vi "RRTPlan.vi"(8 "Initial Pos x,y":dbl[](array[numeric]), 9 "Dest x,y":dbl[](array[numeric]), 10 "IA State":T3={"our_robots"=[], "enemy_robots"=[], "balls"=[], "geometry"={"field_length"=0, "field_width"=0, "goal_width"=0, "goal_depth"=0, "center_circle_radius"=0, "defense_width"=0, "defense_depth"=0, "free_kick_from_defense_dist"=0, "penalty_spot_from_field_line_dist"=0, "penalty_line_from_spot_dist"=0, "half_moon_depth"=0, "half_moon_width"=0}, "IA Judge"={"stage"="", "command"="", "our_goalie_id"=0.0, "enemy_goalie_id"=0.0, "command enum"=enum."Halt", "Time"=enum."Azul"}, "Received Timestamp"=timestamp(0 s since 1904-01-01), "Events"={"Touch"=FALSE, "id touch"=0.0, "Ball out of \nVision"=FALSE, "Ball inside \nGoalie area"=FALSE, "Robot not responding"=FALSE, "Robots responding status"=[1.0, 1.0, 1.0, 1.0, 1.0, 1.0], "Enemy Ball \nPossession"=FALSE, "Id ini Possession"=0.0, "Ball Possesion"=FALSE, "Id Possesion"=0.0, "Ball at\nour goal side"=FALSE, "Ball at\ntouchline"=FALSE, "Ball at\nenemy goal side"=FALSE}}, 11 "Robot":T4={"id"=0, "function"=enum."Attacker", "x"=0.0, "y"=0.0, "orientation"=0.0, "v_tangent"=0.0, "v_normal"=0.0, "v_ang"=0.0, "kick_x"=0.0, "kick_z"=0.0, "dribble"=FALSE, "Timestamp"=timestamp(0 s since 1904-01-01), "estimatives"={"est_v_tangent"=0.0, "est_v_normal"=0.0, "est_vx"=0.0, "est_vy"=0.0, "Pos Robot Est"=[]}, "dest_x_kick"=0.0, "dest_y_kick"=0.0, "Gap Coord"=[], "States"=enum."GoToTangent", "Path "=[], "Path  Smooth"=[], "Dest"=[]}) -> (0 "Path":dbl[][](array[numeric]), 1 "Smooth Path":dbl[][](array[numeric]))   [LabVIEW 2018]
uses:
  Core/AI Robot.ctl
  Intel/Functions Enum.ctl
  Intel/AttackerStates.ctl
  PathDests.ctl
  PathDest.ctl
  Core/AI Input.ctl
  Core/AI Ball.ctl
  Core/Field Size.ctl
  Core/AI Judge.ctl
  Intel/Command Enum.ctl
  Util/Events/Events.ctl
  kD-tree/KD-Tree.ctl
  kD-tree/Node.ctl
  <vilib>/Analysis/_algsub.llb/Real Vector Norm.vi
  <vilib>/Analysis/NI_AALPro.lvlib
panel:
  out "New KD-Tree":T1
  out "x > y? 2":bool
  out "Modulo":dbl
  in  "WayPointProb":dbl=0.6 format="%#_13g"
  in  "GoalProb":dbl=0.1 format="%#_13g"
  in  "Step":dbl=80.0
  out "Elapsed Time (s)":dbl
  out "Time has Elapsed":bool
  in  "threshold":dbl=80.0
  out "Goal":dbl[](array[numeric])
  out "Initial State":dbl[](array[numeric])
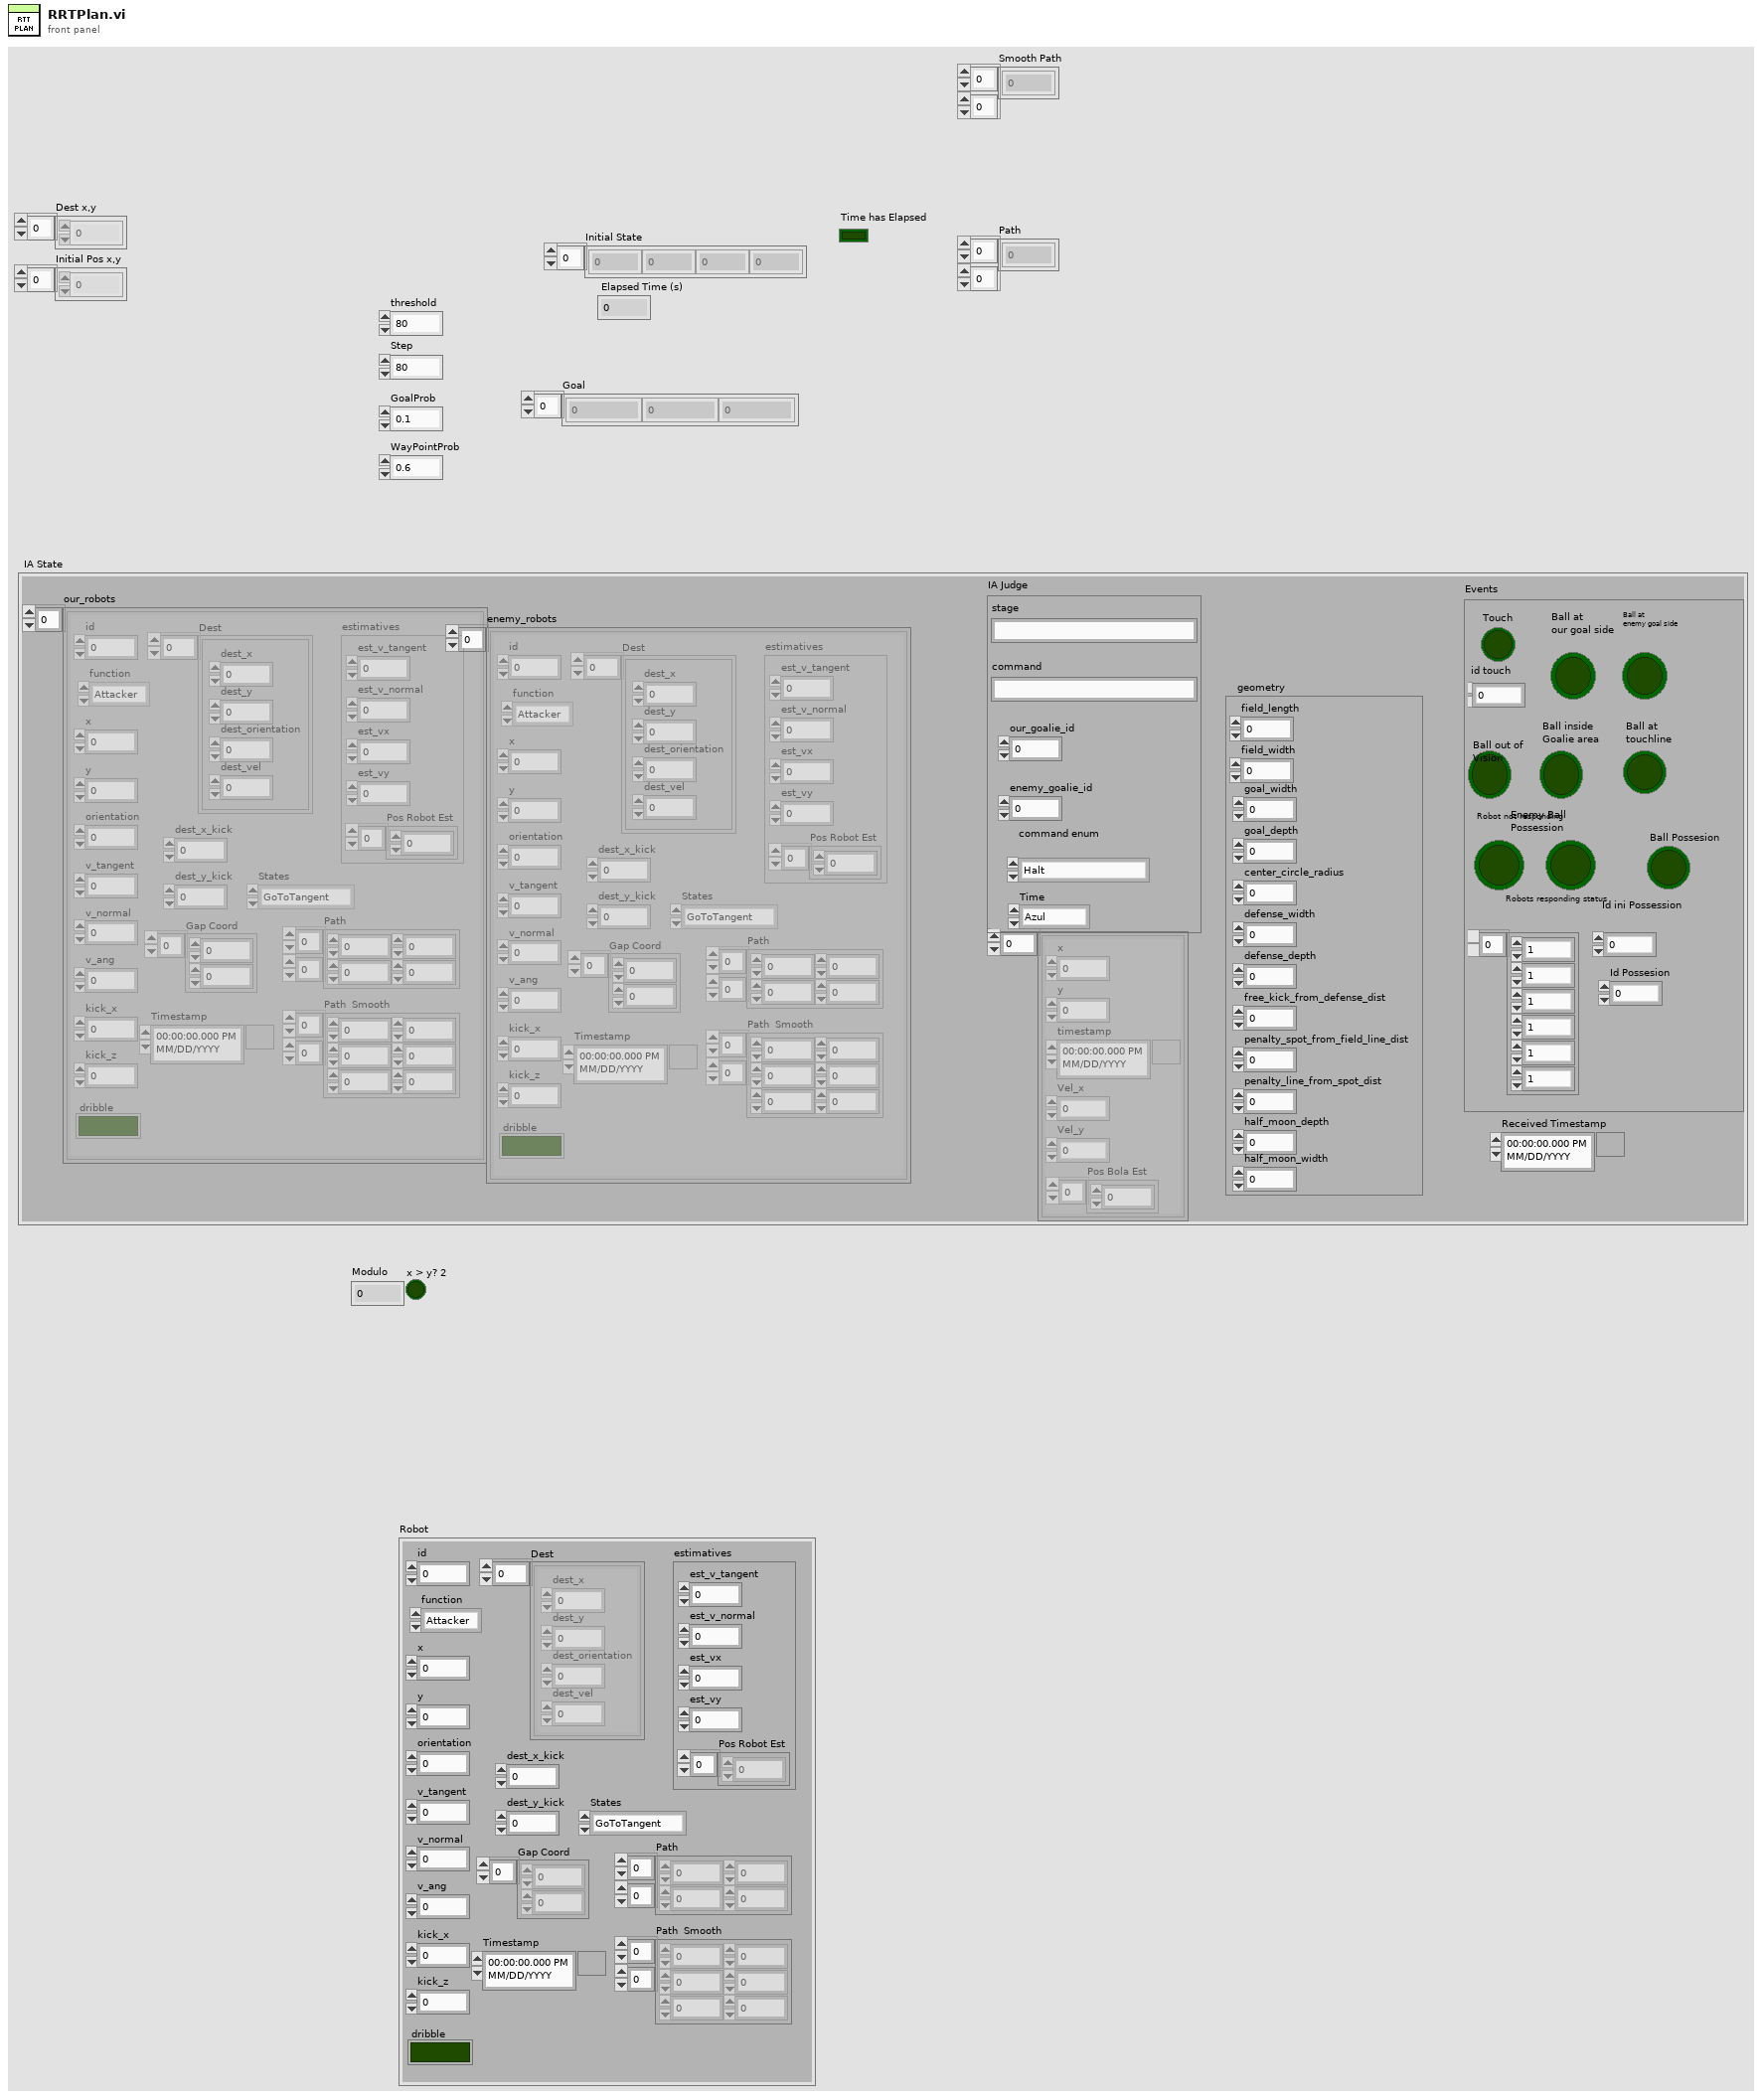
[diagram p1: front panel]
types:
  T1 = typedef "KD-Tree.ctl" = T2[]
  T2 = typedef "Node.ctl" = cluster{"axis":enum16{"null", "x", "y"}, "value":dbl, "left":dbl, "right":dbl, "Point":dbl[]}
  T3 = typedef "AI Input.ctl" = cluster{"our_robots":T4[], "enemy_robots":T4[], "balls":T9[], "geometry":T10, "IA Judge":T11, "Received Timestamp":timestamp, "Events":T13}
  T4 = typedef "AI Robot.ctl" = cluster{"id":u32, "function":T5, "x":dbl, "y":dbl, "orientation":dbl, "v_tangent":dbl, "v_normal":dbl, "v_ang":dbl, "kick_x":dbl, "kick_z":dbl, "dribble":bool, "Timestamp":timestamp, "estimatives":cluster{"est_v_tangent":dbl, "est_v_normal":dbl, "est_vx":dbl, "est_vy":dbl, "Pos Robot Est":dbl[]}, "dest_x_kick":dbl, "dest_y_kick":dbl, "Gap Coord":dbl[], "States":T6, "Path ":dbl[][], "Path  Smooth":dbl[][], "Dest":T7}
  T5 = typedef "Functions Enum.ctl" = enum16{"Attacker", "Goalie", "Defender", "Striker", "Goto 0", "Dummy", "Kicker", "ZigZag"}
  T6 = typedef "AttackerStates.ctl" = enum16{"Pass", "GoToTangent", "BallGetting", "GoToKick", "Rotate anti-clockwise", "Rotate Clockwise", ""}
  T7 = typedef "PathDests.ctl" = T8[]
  T8 = typedef "PathDest.ctl" = cluster{"dest_x":dbl, "dest_y":dbl, "dest_orientation":dbl, "dest_vel":dbl}
  T9 = typedef "AI Ball.ctl" = cluster{"x":dbl, "y":dbl, "timestamp":timestamp, "Vel_x":dbl, "Vel_y":dbl, "Pos Bola Est":dbl[]}
  T10 = typedef "Field Size.ctl" = cluster{"field_length":u32, "field_width":u32, "goal_width":u32, "goal_depth":u32, "center_circle_radius":u32, "defense_width":u32, "defense_depth":u32, "free_kick_from_defense_dist":u32, "penalty_spot_from_field_line_dist":u32, "penalty_line_from_spot_dist":u32, "half_moon_depth":u32, "half_moon_width":u32}
  T11 = typedef "AI Judge.ctl" = cluster{"stage":string, "command":string, "our_goalie_id":dbl, "enemy_goalie_id":dbl, "command enum":T12, "Time":enum16{"Azul", "Amarelo"}}
  T12 = typedef "Command Enum.ctl" = enum16{"Halt", "Stop", "Force Start", "PKA Normal Start", "Prepare Kickoff Ally", "PKE Normal Start", "Prepare Kickoff Enemy", "Prepare Penalty Ally", "PPA Normal Start", "Prepare Penalty Enemy", "PPE Normal Start", "Ball Placement Enemy Up", "Ball Placement Enemy Down", "Ball Placement Ally Up", "Ball Placement Ally Mid", "Ball Placement Ally Down", "Indirect Free Enemy", "Indirect Free Ally", "Timeout Enemy", "Timeout Ally", "Goal Enemy", "Goal Ally", "Normal Half Time", "Extra Time Break", "Extra Half Time", "None", "Post Game"}
  T13 = typedef "Events.ctl" = cluster{"Touch":bool, "id touch":dbl, "Ball out of \nVision":bool, "Ball inside \nGoalie area":bool, "Robot not responding":bool, "Robots responding status":dbl[], "Enemy Ball \nPossession":bool, "Id ini Possession":dbl, "Ball Possesion":bool, "Id Possesion":dbl, "Ball at\nour goal side":bool, "Ball at\ntouchline":bool, "Ball at\nenemy goal side":bool}
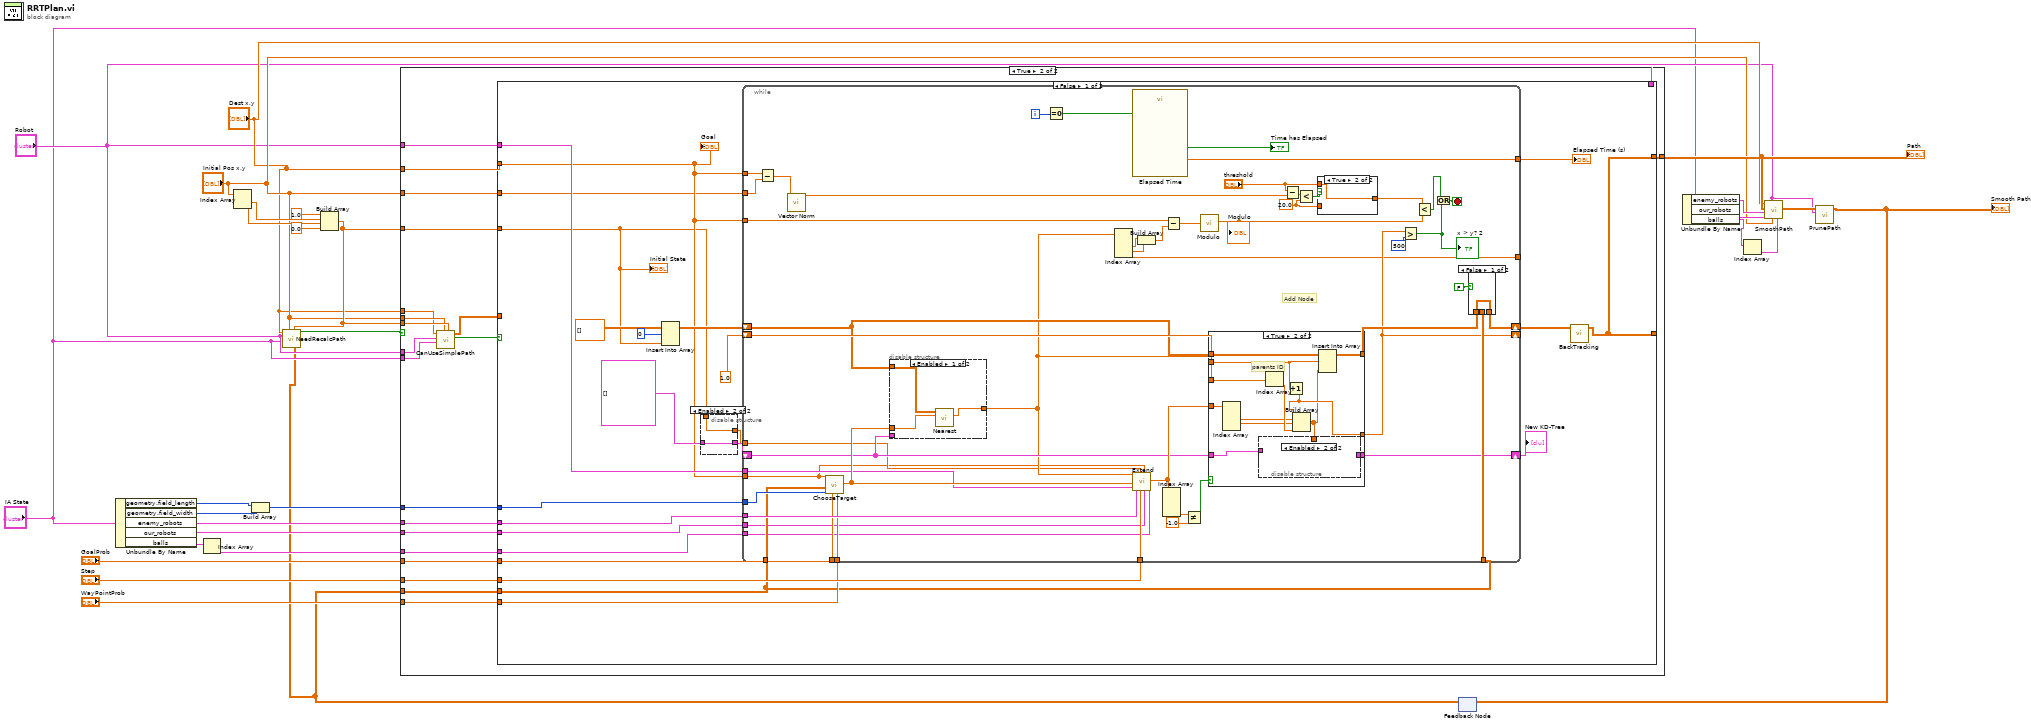
[diagram p0: block diagram]
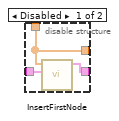
[diagram p3: hidden frame]
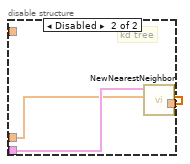
[diagram p4: hidden frame]
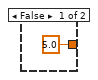
[diagram p5: hidden frame]
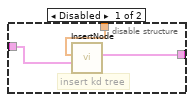
[diagram p8: hidden frame]
diagram:
  n1 = Unbundle By Name("IA State") -> ("geometry.field_length"=w28:u32, "geometry.field_width"=w27:u32, "enemy_robots"=w22:T4[], "our_robots"=w19:T4[], "balls"=w9:T9[])
  n2 = Index Array(array=w9) -> (element=w8:T9)  [unwired: 1 in]
  n3 = Index Array(array="Initial Pos x,y") -> (element #1=w18:dbl, element #2=w17:dbl)  [unwired: 2 in]
  n4 = Build Array(w28, w27) -> (w26:u32[])
  n5 = Build Array(1.0 ("element"), w18, w17, 0.0 ("element")) -> (w6:dbl[])
  n6 = feedback #1() -> (w1:dbl[][])  [unwired: 1 in]
  n7 = call "NeedRecalcPath.vi"("SmoothPath"=w1, "Initial State"=w6, "Pos x,y"="Initial Pos x,y", "IA State"="IA State", "Robot"="Robot", "Dest x,y"="Dest x,y") -> ("Boolean"=w7:bool)  [unwired: 5 in]
  n8 = case shown="True" w7 {
    tunnel: w26 -> [_ w49]
    tunnel: "Step" -> [_ w48]
    tunnel: "GoalProb" -> [_ w47]
    tunnel: "WayPointProb" -> [_ w46]
    tunnel: w22 -> [_ w45]
    tunnel: w6 -> [_ w44]
    tunnel: w1 -> [w29 w43]
    tunnel: w19 -> [_ w42]
    tunnel: [w29 w41] -> w14
    tunnel: "Dest x,y" -> [_ w40]
    tunnel: "Initial Pos x,y" -> [_ w39]
    tunnel: "Robot" -> [_ w38]
    tunnel: w8 -> [_ w37]
    tunnel: w6 -> [_ w36]
    tunnel: "Initial Pos x,y" -> [_ w35]
    tunnel: "Dest x,y" -> [_ w34]
    tunnel: "Robot" -> [_ w33]
    tunnel: "IA State" -> [_ w32]
    frame False {
    }
    frame True {
      n9 = call "CanUseSimplePath.vi"("Initial State"=w36, "Pos x,y"=w35, "IA State"=w32, "Robot"=w33, "Dest x,y"=w34) -> (2:"Simple Path"=w30:bool, 3:"Simple Path"=w31:dbl[][])  [unwired: 5 in]
      n10 = case shown="False" w30 {
        tunnel: w49 -> [w62 _]
        tunnel: w48 -> [w69 _]
        tunnel: w38 -> [w57 _]
        tunnel: w47 -> [w67 _]
        tunnel: w46 -> [w66 _]
        tunnel: w45 -> [w65 _]
        tunnel: w43 -> [w64 _]
        tunnel: [w55 w156] -> w41
        tunnel: w38 -> [_ _]
        tunnel: [w55 w156] -> _
        tunnel: w40 -> [w54 _]
        tunnel: w39 -> [w53 _]
        tunnel: w44 -> [w52 _]
        tunnel: w42 -> [w51 _]
        tunnel: w37 -> [w50 _]
        tunnel: w31 -> [_ w156]
        frame False {
          n11 = Insert Into Array(array=dbl[][] [] ("Pontos"), index (row)=0, new element=w52) -> (w70:dbl[][])  [unwired: 1 in]
          n12 = disable-structure shown="Enabled" {
            disable-tunnel: [w75 w77] -> w60
            disable-tunnel: T1 [] ("New KD-Tree") -> [w74 w77]
            disable-tunnel: w52 -> [w73 w76]
            disable-tunnel: [w73 w76] -> w56
            frame Disabled {
              n13 = call "InsertFirstNode.vi"("New KD-Tree in"=w74, "Tree"=w73) -> ("New KD-Tree out"=w75:T1)  [unwired: 9 in]
            }
            frame Enabled {
            }
          }
          n14 = while {
            tunnel: w54 -> [w126]
            tunnel: w54 -> [w81]
            tunnel: w62 -> [w123]
            shift-right: [w107] -> w63
            shift-left: w70 -> [w106]
            tunnel: w65 -> [w121]
            tunnel: w69 -> [w120]
            shift-right: [w103] -> _
            shift-left: 1.0 -> [w111]
            tunnel: w64 -> [w110]
            tunnel: w64 -> [w109]
            tunnel: w67 -> [w101]
            tunnel: w66 -> [w100]
            tunnel: [w97] -> _
            tunnel: w54 -> [w96]
            shift-right: [w89] -> w61
            shift-left: w60 -> [w88]
            tunnel: [w86] -> w58
            tunnel: w57 -> [w83]
            tunnel: w56 -> [w82]
            tunnel: w53 -> [w80]
            tunnel: w51 -> [w79]
            tunnel: w50 -> [w78]
            i -> [w85]
            stop <- w115 stop-if-true
            w90 = 20.0 ("y")
            # "Add Node"
            n15 = Subtract(x=w96, y=w80) -> (x-y=w95:dbl[])
            n16 = call-poly <vilib>:"Vector Norm.vi"("Input Vector"=w95) -> ("norm"=w93:dbl)  [unwired: 9 in, 1 out]
            n17 = call "ChooseTarget.vi"("WayPointProb"=w100, "GoalProb"=w101, "Field Geometry"=w123, "WayPointCache"=w110, "Goal"=w81) -> ("Target"=w122:dbl[])  [unwired: 6 in]
            n18 = disable-structure shown="Enabled" {
              disable-tunnel: w122 -> [w130 w132]
              disable-tunnel: w106 -> [w129 _]
              disable-tunnel: w88 -> [_ w133]
              disable-tunnel: [w128 w131] -> w87
              frame Enabled {
                n19 = call "Nearest.vi"("Target"=w130, "Pontos"=w129) -> ("Nearest"=w128:dbl[])  [unwired: 9 in]
              }
              frame Disabled {
                # "kd tree"
                n20 = call "NewNearestNeighbor.vi"("q"=w132, "KD-Tree"=w133) -> ("Nearest"=w131:dbl[])  [unwired: 9 in]
              }
            }
            n21 = Equal To 0?(x=w85) -> (x = 0?=w84:bool)
            n22 = Index Array(array=w87) -> (element #2=w114:dbl, element #3=w113:dbl, element #4=w97:dbl)  [unwired: 4 in, 1 out]
            n23 = call "Elapsed Time"("Auto Reset"=w84) -> ("Elapsed Time (s)"=w86:dbl, "Time has Elapsed"=→"Time has Elapsed":bool)  [unwired: 11 in, 6 out]
            n24 = call "Extend.vi"("Ball"=w78, "our_robots"=w79, "Goal"=w81, "Step"=w120, "Initial State"=w82, "enemy_robots"=w121, "Robot in"=w83, "Target"=w122, "Nearest"=w87) -> ("New State"=w116:dbl[])  [unwired: 2 in]
            n25 = Build Array(w114, w113) -> (w112:dbl[])
            n26 = Index Array(array=w116) -> (element #4=w119:dbl)  [unwired: 4 in, 3 out]
            n27 = Subtract(x=w126, y=w112) -> (x-y=w127:dbl[])
            n28 = Not Equal?(x=w119, y=-1.0) -> (x != y?=w117:bool)
            n29 = call "Modulo.vi"("2D vector"=w127) -> ("Modulo"=w125:dbl)  [unwired: 10 in]
            "Modulo" <- w125
            n30 = case shown="True" w117 {
              tunnel: w106 -> [w140 w152]
              tunnel: [w140 w148] -> w108
              tunnel: w116 -> [_ w151]
              tunnel: w111 -> [w139 w147]
              tunnel: w87 -> [_ w150]
              tunnel: [w139 w142] -> w103
              tunnel: [w138 w146] -> w89
              tunnel: w88 -> [w138 w145]
              frame False {
              }
              frame True {
                # "parents ID"
                n31 = Index Array(array=w151) -> (element #2=w144:dbl, element #3=w143:dbl)  [unwired: 4 in, 2 out]
                n32 = Index Array(array=w150) -> (element=w149:dbl)  [unwired: 1 in]
                n33 = Increment(x=w147) -> (x+1=w142:dbl)
                n34 = Build Array(w142, w144, w143, w149) -> (w141:dbl[])
                n35 = disable-structure shown="Enabled" {
                  disable-tunnel: [w155 _] -> w146
                  disable-tunnel: w145 -> [w154 _]
                  disable-tunnel: w141 -> [w153 _]
                  frame Disabled {
                    # "insert kd tree"
                    n36 = call "InsertNode.vi"("KD-Tree"=w154, "New Node"=w153) -> ("New KD-Tree"=w155:T1)  [unwired: 9 in]
                  }
                  frame Enabled {
                  }
                }
                n37 = Insert Into Array(array=w152, index (row)=w147, new element=w141) -> (w148:dbl[][])  [unwired: 1 in]
              }
            }
            n38 = Subtract(x="threshold", y=w93) -> (x-y=w91:dbl)
            n39 = Less?(x=w91, y=w90) -> (x < y?=w92:bool)
            n40 = case shown="True" w92 {
              tunnel: [5.0 ("threshold") w135] -> w124
              tunnel: "threshold" -> [_ w135]
              tunnel: w90 -> [_ _]
              frame False {
              }
              frame True {
              }
            }
            n41 = Greater?(x=w103, y=500) -> (0:w98:bool)
            "x > y? 2" <- w98
            n42 = Less?(x=w125, y=w124) -> (x < y?=w99:bool)
            n43 = Or(x=w99, y=w98) -> (x .or. y?=w115:bool)
            n44 = case shown="False" FALSE {
              tunnel: w109 -> [_ w137]
              tunnel: [w136 w137] -> w107
              tunnel: w108 -> [w136 _]
              frame False {
              }
              frame True {
              }
            }
          }
          "New KD-Tree" <- w61
          "Elapsed Time (s)" <- w58
          n45 = call "BackTracking.vi"("Pontos"=w63) -> ("Path"=w55:dbl[][])  [unwired: 9 in, 1 out]
          "Initial State" <- w52
          "Goal" <- w54
        }
        frame True {
        }
      }
    }
  }
  "Path" <- w14
  n46 = Unbundle By Name("IA State") -> ("enemy_robots"=w15:T4[], "our_robots"=w16:T4[], "balls"=w11:T9[])
  n47 = Index Array(array=w11) -> (element=w10:T9)  [unwired: 1 in]
  n48 = call "SmoothPath.vi"("ball"=w10, "Initial State"="Initial Pos x,y", "Robot in"="Robot", "our_robots"=w16, "enemy_robots"=w15, "Path"=w14, "Goal"="Dest x,y") -> ("SmoothPath"=w13:dbl[][])  [unwired: 4 in]
  n49 = call "PrunePath.vi"("Robot in"="Robot", "Path in"=w13) -> ("Path out"=w12:dbl[][])  [unwired: 8 in, 1 out]
  "Smooth Path" <- w12
  n50 = feedback-in #1(w12) -> ()
